vi "AssembleStats.vi"(9 "ExcessiveConeFraction":dbl, 10 "ValidFraction":dbl, 11 "VmagUVWCone":dbl[][](array[numeric])) -> (1 "Plug in titles":string[](array[string])=["\\overline{V_{mag}}", "\\sigma^2(V_{mag})", "\\overline{U}", "\\sigma^2(U)", "\\overline{V}", "\\sigma^2(V)", "\\overline{W}", "\\sigma^2(W)", "\\overline{u'v'}", "\\overline{v'w'}", "\\overline{u'w'}", "\\overline{\\theta}", "\\sigma^2(\\theta)", "GoodFraction", "ExceededConeFraction"], 3 "StatsArray":dbl[](array[numeric]))   [LabVIEW 2013]
uses:
  <vilib>/Analysis/NI_AALBase.lvlib
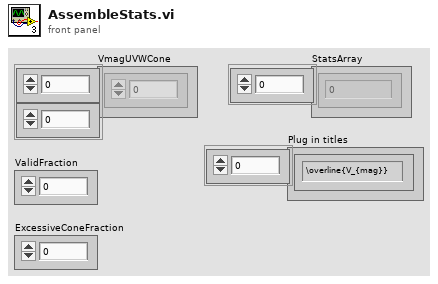
[diagram p1: front panel]
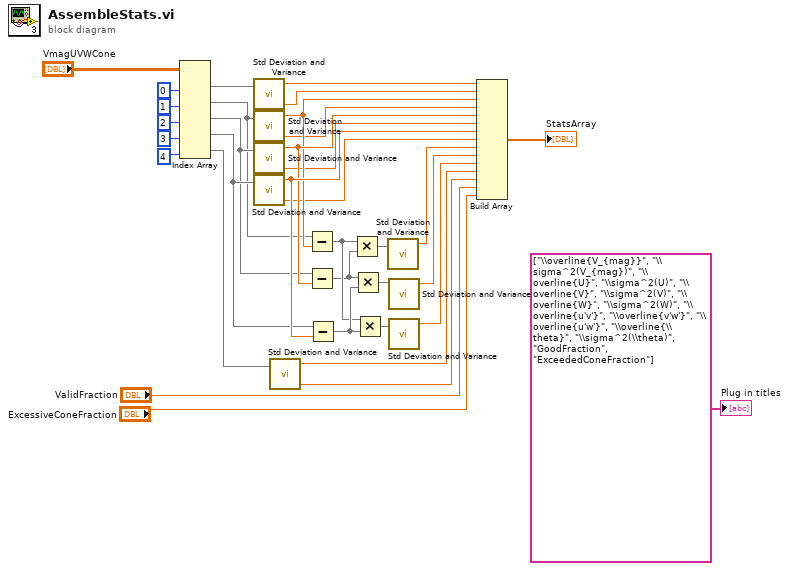
[diagram p0: block diagram]
diagram:
  n1 = Index Array(array="VmagUVWCone", index (col) #1=0 ("disabled index (col)"), index (col) #2=1 ("index (col)"), index (col) #3=2 ("index (col)"), index (col) #4=3 ("index (col)"), index (col) #5=4 ("index (col)")) -> (element #1=w2:dbl[], element #2=w13:dbl[], element #3=w16:dbl[], element #4=w18:dbl[], element #5=w30:dbl[])  [unwired: 5 in]
  n2 = call <vilib>:"Std Deviation and Variance.vi"("X"=w2) -> ("mean"=w14:dbl, "variance"=w8:dbl)  [unwired: 1 in, 1 out]
  n3 = call <vilib>:"Std Deviation and Variance.vi"("X"=w13) -> ("mean"=w15:dbl, "variance"=w9:dbl)  [unwired: 1 in, 1 out]
  n4 = call <vilib>:"Std Deviation and Variance.vi"("X"=w16) -> ("mean"=w17:dbl, "variance"=w10:dbl)  [unwired: 1 in, 1 out]
  n5 = call <vilib>:"Std Deviation and Variance.vi"("X"=w18) -> ("mean"=w19:dbl, "variance"=w11:dbl)  [unwired: 1 in, 1 out]
  n6 = call <vilib>:"Std Deviation and Variance.vi"("X"=w30) -> ("mean"=w31:dbl, "variance"=w32:dbl)  [unwired: 1 in, 1 out]
  n7 = Subtract(x=w13, y=w15) -> (x-y=w22:dbl[])
  n8 = Subtract(x=w16, y=w17) -> (x-y=w21:dbl[])
  n9 = Subtract(x=w18, y=w19) -> (x-y=w23:dbl[])
  n10 = Multiply(x=w22, y=w21) -> (x*y=w20:dbl[])
  n11 = Multiply(x=w21, y=w23) -> (x*y=w25:dbl[])
  n12 = Multiply(x=w22, y=w23) -> (x*y=w24:dbl[])
  n13 = call <vilib>:"Std Deviation and Variance.vi"("X"=w20) -> ("mean"=w26:dbl)  [unwired: 1 in, 2 out]
  n14 = call <vilib>:"Std Deviation and Variance.vi"("X"=w25) -> ("mean"=w27:dbl)  [unwired: 1 in, 2 out]
  n15 = call <vilib>:"Std Deviation and Variance.vi"("X"=w24) -> ("mean"=w28:dbl)  [unwired: 1 in, 2 out]
  n16 = Build Array(w14, w8, w15, w9, w17, w10, w19, w11, w26, w27, w28, w31, w32, "ValidFraction", "ExcessiveConeFraction") -> (→"StatsArray":dbl[])
  "Plug in titles" <- string[] ["\\overline{V_{mag}}", "\\sigma^2(V_{mag})", "\\overline{U}", "\\sigma^2(U)", "\\overline{V}", "\\sigma^2(V)", "\\overline{W}", "\\sigma^2(W)", "\\overline{u'v'}", "\\overline{v'w'}", "\\overline{u'w'}", "\\overline{\\theta}", "\\sigma^2(\\theta)", "GoodFraction", "ExceededConeFraction"] ("Plug in titles")
